vi "assert.vi"(10 "mustBeTrue":bool) -> ()   [LabVIEW 2013]
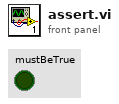
[diagram p1: front panel]
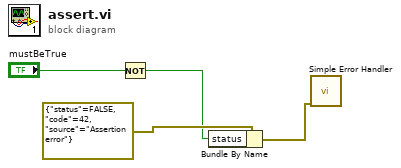
[diagram p0: block diagram]
diagram:
  n1 = Not(x="mustBeTrue") -> (.not. x?=w1:bool)
  n2 = Bundle By Name(cluster=errorcluster {"status"=FALSE, "code"=42, "source"="Assertion error"} ("error constant"), "status"=w1) -> (w2:errorcluster)
  n3 = call <vilib>:"Simple Error Handler.vi"("error in (no error)"=w2) -> ()  [unwired: 4 in, 5 out]
